vi "Create Custom Char.vi"(7 "Location 0-7":u8, 8 "error in (no error)":errorcluster, 9 "Char":T1=[[FALSE, FALSE, FALSE, FALSE, FALSE], [FALSE, FALSE, FALSE, FALSE, FALSE], [FALSE, FALSE, FALSE, FALSE, FALSE], [FALSE, FALSE, FALSE, FALSE, FALSE], [FALSE, FALSE, FALSE, FALSE, FALSE], [FALSE, FALSE, FALSE, FALSE, FALSE], [FALSE, FALSE, FALSE, FALSE, FALSE], [FALSE, FALSE, FALSE, FALSE, FALSE]], 10 "VISA resource name in":refnum<visa-resource-name>, 11 "LCD-I2C in":refnum<class "LCD-I2C.lvclass">) -> (0 "error out":errorcluster, 2 "VISA resource name":refnum<visa-resource-name>, 3 "LCD-I2C out":refnum<class "LCD-I2C.lvclass">)   [LabVIEW 2023, in "CTI-Visa-DeviceLib.lvlib" / "LCD-I2C.lvclass"]
uses:
  LCD-I2C.lvclass
  Custom Char.ctl
  Command.ctl
  Mode.ctl
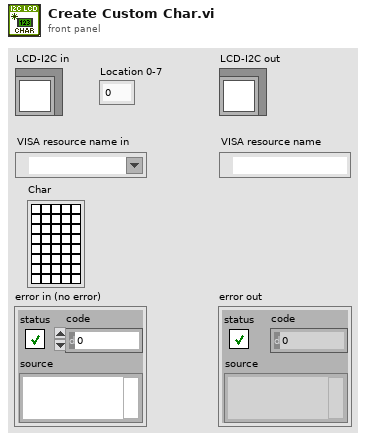
[diagram p1: front panel]
types:
  T1 = typedef "CTI-Visa-DeviceLib.lvlib/LCD-I2C.lvclass/Custom Char.ctl" = bool[][]
  T2 = typedef "CTI-Visa-DeviceLib.lvlib/LCD-I2C.lvclass/Command.ctl" = enum16{"Clear Display", "Return Home", "Entry Mode Set", "Display Control", "Cursor Shift", "Function Set", "Set CGRAM Addr", "Set DDRAM Addr"}
  T3 = typedef "CTI-Visa-DeviceLib.lvlib/LCD-I2C.lvclass/Mode.ctl" = enum8{"Command", "Character"}
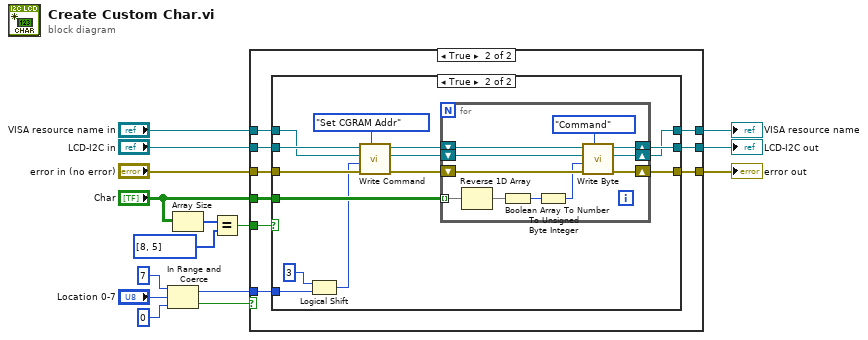
[diagram p0: block diagram]
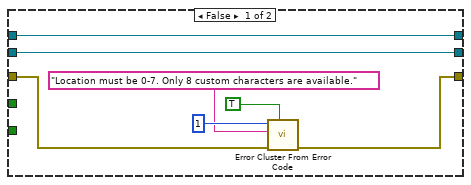
[diagram p2: hidden frame]
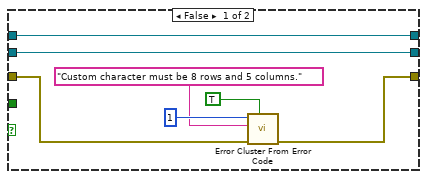
[diagram p3: hidden frame]
diagram:
  n1 = In Range and Coerce(upper limit=u8 7 ("lower limit"), x="Location 0-7", lower limit=u8 0) -> (coerced(x)=w11:u8, In Range?=w12:bool)
  n2 = Array Size(array="Char") -> (size(s)=w7:i32[])
  n3 = Equal?(x=w7, y=i32[] [8, 5]) -> (x = y?=w5:bool)
  n4 = case shown="True" w12 {
    tunnel: w11 -> [_ w27]
    tunnel: "LCD-I2C in" -> [w21 w29]
    tunnel: "error in (no error)" -> [w17 w28]
    tunnel: "Char" -> [_ w31]
    tunnel: w5 -> [_ w30]
    tunnel: "VISA resource name in" -> [w22 w26]
    tunnel: [w22 w25] -> w3
    tunnel: [w21 w24] -> w2
    tunnel: [w16 w23] -> w1
    frame False {
      n5 = call <vilib>:"Error Cluster From Error Code.vi"("show call chain? (False)"=TRUE, "error in (no error)"=w17, "error message (\"\")"="Location must be 0-7. Only 8 custom characters are available.", "error code (0)"=1) -> ("error out"=w16:errorcluster)  [unwired: 5 in]
    }
    frame True {
      n6 = case shown="True" w30 {
        tunnel: w31 -> [_ w52]
        tunnel: w29 -> [w37 w49]
        tunnel: w28 -> [w33 w51]
        tunnel: w27 -> [_ w44]
        tunnel: w26 -> [w38 w45]
        tunnel: [w38 w39] -> w25
        tunnel: [w37 w42] -> w24
        tunnel: [w32 w40] -> w23
        frame False {
          n7 = call <vilib>:"Error Cluster From Error Code.vi"("show call chain? (False)"=TRUE, "error in (no error)"=w33, "error message (\"\")"="Custom character must be 8 rows and 5 columns.", "error code (0)"=1) -> ("error out"=w32:errorcluster)  [unwired: 5 in]
        }
        frame True {
          n8 = Logical Shift(y=i16 3, x=w44) -> (x << y=w41:u8)
          n9 = call "Write Command.vi"("Command"=Command."Set CGRAM Addr", "error in (no error)"=w51, "Value"=w41, "VISA resource name in"=w45, "LCD-I2C in"=w49) -> ("error out"=w50:errorcluster, "VISA resource name"=w46:refnum<visa-resource-name>, "LCD-I2C out"=w48:refnum<class "LCD-I2C.lvclass">)  [unwired: 4 in]
          n10 = for {
            tunnel: w52 -> [w63] mode=indexing
            shift-right: [w54] -> w40
            shift-left: w50 -> [w58]
            shift-right: [w56] -> w42
            shift-left: w48 -> [w60]
            shift-right: [w55] -> w39
            shift-left: w46 -> [w59]
            n11 = Reverse 1D Array(array=w63) -> (reversed array=w53:bool[])
            n12 = Boolean Array To Number(Boolean array=w53) -> (number=w62:u32)
            n13 = To Unsigned Byte Integer(number=w62) -> (unsigned 8bit integer=w57:u8)
            n14 = call "Write Byte.vi"("Mode (Command)"=Mode."Command", "error in (no error)"=w58, "Value"=w57, "VISA resource name in"=w59, "LCD-I2C in"=w60) -> ("error out"=w54:errorcluster, "VISA resource name"=w55:refnum<visa-resource-name>, "LCD-I2C out"=w56:refnum<class "LCD-I2C.lvclass">)  [unwired: 4 in]
          }
        }
      }
    }
  }
  "error out" <- w1
  "LCD-I2C out" <- w2
  "VISA resource name" <- w3
